vi "main_analysis.vi"() -> ()   [LabVIEW 2020]
uses:
  <vilib>/Utility/file.llb/Read Delimited Spreadsheet (string).vi
panel:
  out "appended array":dbl[][](array[numeric])
  out "deleted portion":string[](array[string])
  out "XY Graph":cluster{dbl[], dbl[]}[](graph)
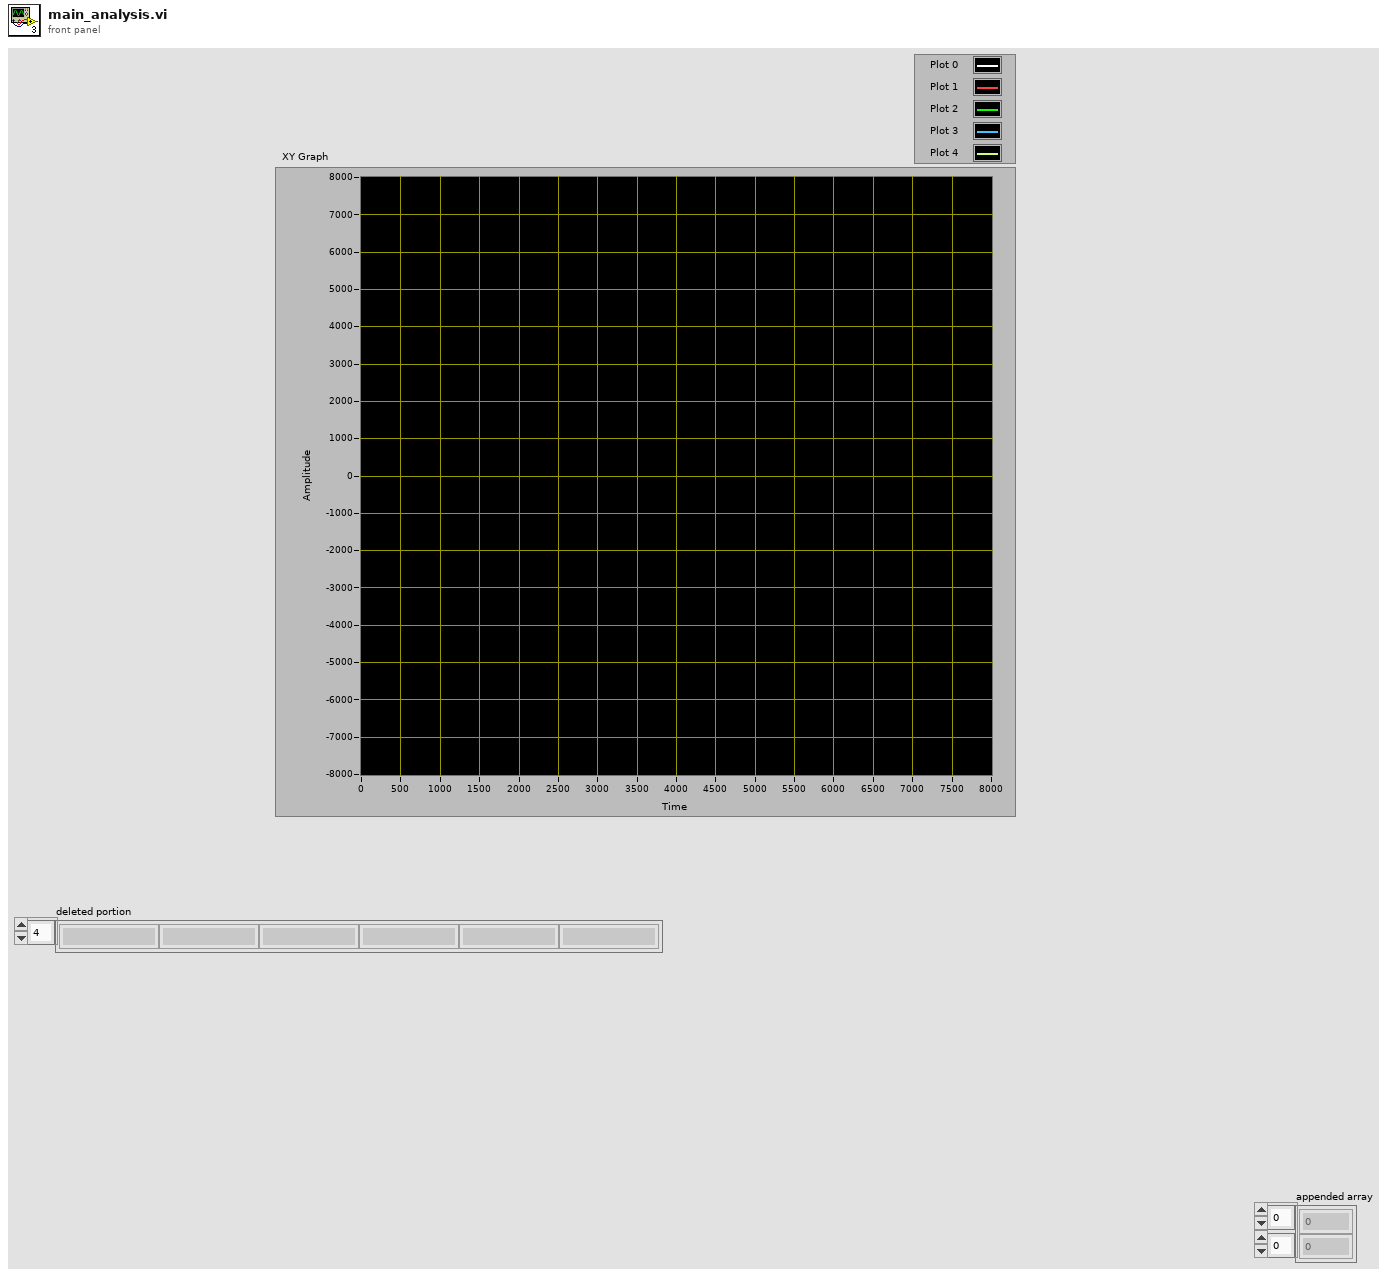
[diagram p1: front panel]
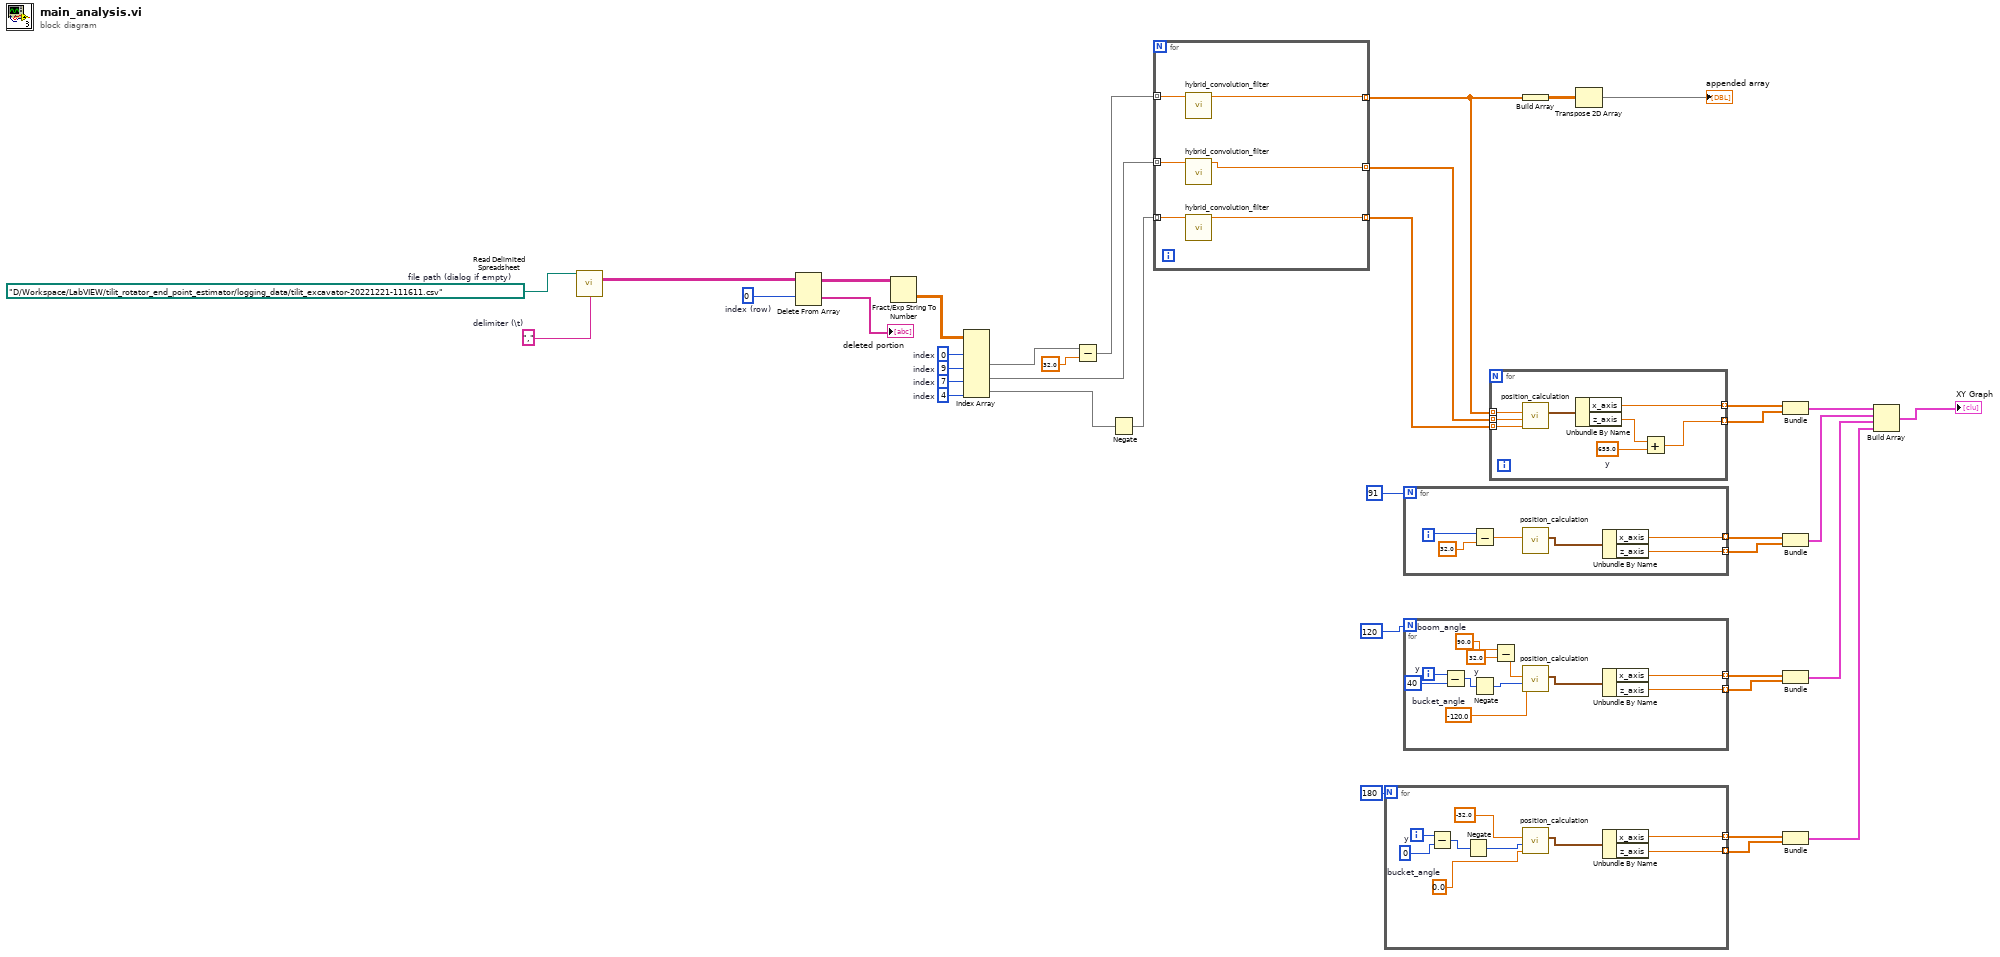
[diagram p0: block diagram]
diagram:
  w23 = 0  # index
  w28 = 4  # index
  w29 = 7  # index
  w31 = 9  # index
  w35 = 0  # index (row)
  w37 = ","  # delimiter (\t)
  w38 = path "D:/Workspace/LabVIEW/tilit_rotator_end_point_estimator/logging_data/tilit_excavator-20221221-111611.csv"  # file path (dialog if empty)
  n1 = call-poly <vilib>:"Read Delimited Spreadsheet.vi"("file path (dialog if empty)"=w38, "delimiter (\\t)"=w37) -> ("all rows"=w36:string[][])  [unwired: 8 in, 5 out]
  n2 = Delete From Array "Delete From Array"(array=w36, index (row)=w35) -> (deleted portion=→"deleted portion":string[], array with subset deleted=w33:string[][])  [unwired: 2 in]
  n3 = Fract/Exp String To Number(string=w33) -> (number=w32:dbl[][])  [unwired: 3 in, 1 out]
  n4 = Index Array "Index Array"(array=w32, index (col) #1=w23, index (col) #2=w31, index (col) #3=w29, index (col) #4=w28) -> (element #2=w22:dbl[], element #3=w17:dbl[], element #4=w27:dbl[])  [unwired: 4 in, 1 out]
  n5 = Subtract(x=w22, y=32.0) -> (x-y=w19:dbl[])
  n6 = Negate(x=w27) -> (-x=w15:dbl[])
  n7 = for {
    tunnel: w19 -> [w44] mode=indexing
    tunnel: [w43] -> w18 mode=indexing
    tunnel: w17 -> [w42] mode=indexing
    tunnel: [w41] -> w16 mode=indexing
    tunnel: w15 -> [w40] mode=indexing
    tunnel: [w39] -> w14 mode=indexing
    n8 = call "hybrid_convolution_filter.vi"("input"=w44) -> ("output"=w43:dbl)  [unwired: 10 in]
    n9 = call "hybrid_convolution_filter.vi"("input"=w42) -> ("output"=w41:dbl)  [unwired: 10 in]
    n10 = call "hybrid_convolution_filter.vi"("input"=w40) -> ("output"=w39:dbl)  [unwired: 10 in]
  }
  n11 = for {
    N: 180 -> [_]
    tunnel: [w52] -> w3 mode=indexing
    tunnel: [w51] -> w2 mode=indexing
    i -> [w47]
    w45 = 0  # y
    w48 = 0.0  # bucket_angle
    n12 = Subtract(x=w47, y=w45) -> (x-y=w46:i32)
    n13 = Negate(x=w46) -> (-x=w49:i32)
    n14 = call "position_calculation.vi"("bucket_angle"=w48, "arm_angle"=w49, "boom_angle"=-32.0) -> ("end_point"=w53:cluster{"x_axis":dbl, "z_axis":dbl})  [unwired: 8 in]
    n15 = Unbundle By Name(w53) -> ("x_axis"=w52:dbl, "z_axis"=w51:dbl)
  }
  n16 = for {
    N: 91 -> [_]
    tunnel: [w55] -> w12 mode=indexing
    tunnel: [w54] -> w11 mode=indexing
    i -> [w58]
    n17 = Subtract(x=w58, y=32.0) -> (x-y=w57:dbl)
    n18 = call "position_calculation.vi"("boom_angle"=w57) -> ("end_point"=w56:cluster{"x_axis":dbl, "z_axis":dbl})  [unwired: 10 in]
    n19 = Unbundle By Name(w56) -> ("x_axis"=w55:dbl, "z_axis"=w54:dbl)
  }
  n20 = for {
    N: 120 -> [_]
    tunnel: [w69] -> w7 mode=indexing
    tunnel: [w68] -> w6 mode=indexing
    i -> [w62]
    w61 = 40  # y
    w63 = -120.0  # bucket_angle
    w66 = 32.0  # y
    w67 = 90.0  # boom_angle
    n21 = Subtract(x=w62, y=w61) -> (x-y=w60:i32)
    n22 = Negate(x=w60) -> (-x=w64:i32)
    n23 = Subtract(x=w67, y=w66) -> (x-y=w65:dbl)
    n24 = call "position_calculation.vi"("bucket_angle"=w63, "arm_angle"=w64, "boom_angle"=w65) -> ("end_point"=w70:cluster{"x_axis":dbl, "z_axis":dbl})  [unwired: 8 in]
    n25 = Unbundle By Name(w70) -> ("x_axis"=w69:dbl, "z_axis"=w68:dbl)
  }
  n26 = for {
    tunnel: w18 -> [w71] mode=indexing
    tunnel: w16 -> [w77] mode=indexing
    tunnel: w14 -> [w76] mode=indexing
    tunnel: [w75] -> w26 mode=indexing
    tunnel: [w72] -> w25 mode=indexing
    w73 = 655.0  # y
    n27 = call "position_calculation.vi"("bucket_angle"=w76, "arm_angle"=w77, "boom_angle"=w71) -> ("end_point"=w78:cluster{"x_axis":dbl, "z_axis":dbl})  [unwired: 8 in]
    n28 = Unbundle By Name(w78) -> ("x_axis"=w75:dbl, "z_axis"=w74:dbl)
    n29 = Add(x=w74, y=w73) -> (x+y=w72:dbl)
  }
  n30 = Build Array(w18) -> (w21:dbl[][])
  n31 = Transpose 2D Array(2D array=w21) -> (transposed array=→"appended array":dbl[][])
  n32 = Bundle(w26, w25) -> (w24:cluster{dbl[], dbl[]})  [unwired: 1 in]
  n33 = Bundle(w12, w11) -> (w9:cluster{dbl[], dbl[]})  [unwired: 1 in]
  n34 = Bundle(w7, w6) -> (w5:cluster{dbl[], dbl[]})  [unwired: 1 in]
  n35 = Bundle(w3, w2) -> (w1:cluster{dbl[], dbl[]})  [unwired: 1 in]
  n36 = Build Array(w24, w9, w5, w1) -> (→"XY Graph":cluster{dbl[], dbl[]}[])
